vi "niScope Measure Dead Time.vi"(2 "error in":errorcluster, 3 "min sample rate":dbl=10000000.0 caption="Min. Sample Rate" step=1000000.0 format="%.3p", 4 "resource name":refnum<k15>="DAQ::1" caption="Resource Name") -> (0 "error out":errorcluster {"code" format="%.0x"}, 1 "Observed DeadTime":dbl)   [LabVIEW 2015]
doc: "Example: Measurement Library\n\nRecommended Input Signal: 100 kHz, 8 Vpp, sine wave\n\nDevices Supported: Refer to NI Example Finders\n\nLabVIEW Description:\n\nThis example illustrates fetching scalar measurements from NI-SCOPE, such as period and rise time calculations. \n\nSome common horizontal and vertical parameters are configured for the digitizer. The property node is used to set the reference level units, and the low, middle and high reference levels. For more information about measurement library parameters, see the NI-SCOPE VI Reference Help file. \n\nAfter the Read VI is called to acquire a waveform, the Fetch Measurement Stats VI is used to perform the desired scalar measurement analysis on the waveform. NI-SCOPE keeps a history of each measurement's results, which allows it to retrieve the statistics computed over multiple acquisitions. These statistics include the mean, standard deviation, min, max and number of acquisitions used in the statistics. The statistics are updated once per acquisition when the measurement is fetched. The Clear Stats VI clears this history."
uses:
  <instrlib>/niScope/Controls/niScope vertical coupling.ctl
  <instrlib>/niScope/Controls/niScope trigger source.ctl
  <instrlib>/niScope/Controls/niScope trigger coupling.ctl
  <instrlib>/niScope/Controls/niScope scalar measurement.ctl
  <instrlib>/niScope/Controls/niScope array measurement.ctl
  <instrlib>/niScope/Configure/Trigger/niScope Configure Trigger Edge.vi
  <instrlib>/niScope/Acquire/niScope Multi Read Cluster.vi
  <instrlib>/niScope/Measurements/niScope Multi Fetch Measurement Stats.vi
panel:
  out "Waveform Chart":u32(graph)
  out "x-y 2":u32
  out "x-y":u32
  out "Observed FallTime Ch 1":dbl format="%^.2e"
  out "Observed FallTime Ch 0":dbl format="%^.2e"
  out "Ch 0 - Fall Time":T1 {"scalar result" format="%^.2e"; "mean" format="%^.2e"; "stdev" format="%^.2e"; "min" format="%^.2e"; "max" format="%^.2e"; "num in stats" format="%^.2e"}
  out "Ch 1 - Fall Time":T1 {"scalar result" format="%^.2e"; "mean" format="%^.2e"; "stdev" format="%^.2e"; "min" format="%^.2e"; "max" format="%^.2e"; "num in stats" format="%^.2e"}
  out "Observed RiseTime Ch 1":dbl format="%^.2e"
  out "Observed RiseTime Ch 0":dbl format="%^.2e"
  out "Ch 0 - Rise Time":T1 {"scalar result" format="%^.2e"; "mean" format="%.2e"; "stdev" format="%.2e"; "min" format="%.2e"; "max" format="%.2e"; "num in stats" format="%.2e"}
  out "Ch 1 - Rise Time":T1 {"scalar result" format="%.2e"; "mean" format="%.2e"; "stdev" format="%.2e"; "min" format="%.2e"; "max" format="%.2e"; "num in stats" format="%.2e"}
  out "Fall Time Measurements":T2(array[cluster]) caption="stats" {"max" format="%^.2e"; "min" format="%^.2e"; "stdev" format="%^.2e"; "mean" format="%^.2e"; "scalar result" format="%^.2e"}
  out "Rise Time Measurements":T2(array[cluster]) caption="stats" {"max" format="%^.2e"; "min" format="%^.2e"; "stdev" format="%^.2e"; "mean" format="%^.2e"; "scalar result" format="%^.2e"}
  out "DeadTime Measurements":T2(array[cluster]) caption="stats" {"max" format="%.2p"; "min" format="%.2p"; "stdev" format="%.2p"; "mean" format="%.2p"; "scalar result" format="%.2p"}
  in  "stop":bool
  in  "Reference Level Units":i32(ring)=1 items=["Voltage", "Percentage"]
  in  "high reference":dbl=90.0 caption="High Ref." format="%.3f"
  in  "mid reference":dbl=50.0 caption="Mid Ref." format="%.3f"
  in  "low reference":dbl=10.0 caption="Low Ref." format="%.3f"
  out "Acquisition Graph":T3(graph)=[{"relativeInitialX"=-5.1119996754778185e-05, "xIncrement"=1e-07, "wfm"=[-4.06403104547644, -4.117707957106177, -4.163333331991453, -4.19755236315541, -4.198223324550781, -4.158636602223851, -4.110327381757088, -4.047927971987519, -3.976135102682747, -3.8835424301214516, -3.782898220815696, -3.6815830501145683, -3.539339234295767, -3.39508253429085, -3.226671224052552, -3.067653373349458, -2.8844809124129824, -2.7019794128718786, -2.5087425310048275, -2.302757382625714, -2.0759724309900776, -1.8491874793544412, -1.6351507942308672, -1.382869309571106, -1.1648068560753018, -0.8991061435081065, -0.6682954235002398, -0.4307750895386562, -0.1818484118557535, 0.0603686518734321, 0.3012437928118743, 0.5488285477040336, 0.7796392677119002, 1.03527555934852, 1.2566928198211826, 1.4888454626197927, 1.7015402249526232, 1.9175897942623124, 2.139678016130347, 2.3315729752066545, 2.5456096603302285, 2.701943665451836, 2.904574006854091, 3.036082440346945, 3.202480866399128, 3.3380150682642125, 3.459459080826491, 3.5607742515276186, 3.6681280747870915, 3.7426047896733508, 3.81305573618738, 3.874113223166205, 3.921751482237596, 3.9593253203784116, 3.9794541622395627, 3.9412093627033755, 3.8908872580504976, 3.842578037583735, 3.7748109366511926, 3.698321337578818, 3.6017028966452926, 3.4997167645487934, 3.3742469836142845, 3.225293553841766, 3.083720699418336, 2.9213480417383835, 2.7522657701047137, 2.5382290849811397, 2.3563985468354076, 2.1249168654321693, 1.9196026784484275, 1.692817726812791, 1.4506006630836055, 1.2278414798201993, 0.9809276863234118, 0.7152269737562165, 0.49515163607429713, 0.23079284629784524, 0.00333693326683715, -0.2529703197651543, -0.503909881634172, -0.7575332890846767, -0.9876730476971716, -1.2104322309605777, -1.4519783332943916, -1.7116403933032416, -1.9511736114509404, -2.1538039528531954, -2.404743514722213, -2.569129056588281, -2.7791399733396247, -2.9797574305557646, -3.1602460459107533, -3.3239606263814494, -3.4816365542938, -3.625222292903345, -3.730563231976703, -3.845968591980636, -3.944599917100277, -4.0090122110559605, -4.0774502733838744, -4.127101416641381, -4.175410637108143, -4.20560389989987, -4.180778328271117, -4.14655929710716, -4.092882385477424, -4.0271281687309965, -3.9519804924493656, -3.860058781283442, -3.760085533373058, -3.6332738296478055, -3.497739627782721, -3.352141004987061, -3.1911102700978518, -3.01733126869658, -2.8435522672953084, -2.6496444240328856, -2.4376206230954267, -2.2356612430885434, -2.0122310984297656, -1.792826722143218, -1.5385323532973416, -1.3218118225922808, -1.088988218398299, -0.8521388458320871, -0.6025412067538127, -0.35227260628016666, -0.1281715002260171, 0.10934883373556659, 0.3616303183953278, 0.6051893049152568, 0.83465810213238, 1.1017007374903187, 1.3157374226138927, 1.524406416574493, 1.779371746815741, 1.9612022849614732, 2.187316275201738, 2.3933014235808514, 2.5711061933543533, 2.7509238473139703, 2.940134960808791, 3.0937851203489117, 3.2420675887260586, 3.370892176637426, 3.4862975366413593, 3.596335205482319, 3.69899229897419, 3.773469013860449, 3.831171693862416, 3.885519566887524, 3.926448212005198, 3.960667243169155, 3.964693011541385, 3.924435327819083, 3.880822837119922, 3.8298297710716724, 3.753340171999298, 3.680876341299154, 3.582245016179513, 3.471536385943182, 3.338686029659584, 3.1951002910500392, 3.0280309036024846, 2.863645361736417, 2.6891953989397734, 2.510048706375528, 2.289302407298237, 2.066543224034831, 1.8598871142603457, 1.6431665835552849, 1.383504523546435, 1.1560486105154268, 0.9171863537630998, 0.6608791007311083, 0.4260426123510115, 0.1757740118773654, -0.06375920627033338, -0.28920223511522636, -0.5730189053574577, -0.8105392393190414, -1.0648336081649177, -1.3117474016617052, -1.5600031179492362, -1.778736532840412, -2.0122310984297656, -2.2309645133209415, -2.43493677751394, -2.648302501242142, -2.844894190086052, -3.0320924193947576, -3.1911102700978518, -3.3648892714991234, -3.5245780835975893, -3.6547445942997, -3.766124185931403, -3.8593878198880702, -3.9539933766354807, -4.025786245940253, -4.094895269663539, -4.145888335711788, -4.183462173852604, -4.210971591062844, -4.172726791526657, -4.137165837571956, -4.082817964546848, -4.010354133846704, -3.9338645347743295, -3.8399299394222908, -3.7245245794183575, -3.609790180809796, -3.4608367510372773, -3.313896205450874, -3.144813933817204, -2.971705893811304, -2.78517862589797, -2.5812063617049716, -2.3926662096055225, -2.173261833318975, -1.9538574570324272, -1.7203628914430737, -1.4929069784120657, -1.257399528636597, -1.036653229559306, -0.7883975132717751, -0.549535256519448, -0.31134396116249263, -0.05839151510735974, 0.1610128611791879, 0.4374489560723305, 0.6709435216616839, 0.9037671258556657, 1.1473261123755947, 1.367401450057514, 1.5921735175070353, 1.8290228900732473, 2.0128663124050945, 2.2403222254361026, 2.430875261721667, 2.6408861784730107, 2.8046007589437068, 2.9803926445310935, 3.138739533838816, 3.272931812913157, 3.3990725552430376, 3.5131359924562275, 3.621160777111072, 3.708385758509394, 3.7821915120002814, 3.8472747673513368, 3.8975968720042147, 3.9365126329357736, 3.9707316640997306, 3.9526157064246945, 3.915041868283879, 3.8680745706078596, 3.814397658978123, 3.7345532529288903, 3.650683078507427, 3.5426582938525826, 3.432620625011623, 3.2990993073326536, 3.1608812598860823, 2.999850524996873, 2.831439214758575, 2.637531371496152, 2.453687949164305, 2.2342835728777573, 2.02293073333567, 1.8109069323982112, 1.588147749134805, 1.355995106336195, 1.1117651584208943, 0.8749157858546823, 0.6118989188689739, 0.38175916025647894, 0.11404556350316852, -0.12213284766767174, -0.3851497146533802, -0.6528633114066906, -0.8709257649024948, -1.111800905840937, -1.346637394221034, -1.6210606049280614, -1.8203361393534578, -2.059198396105785, -2.28933815471828, -2.5020329170511104, -2.700637490081135, -2.896558217529673, -3.0750339486985467, -3.2400904519599862, -3.402463109639939, -3.559468076156918, -3.6742024747654796, -3.791620718955528, -3.8909230054705404, -3.9680835659382865, -4.045915087801404, -4.100262960826512, -4.147230258502532, -4.190842749201693, -4.206945822690614, -4.168030061759055, -4.127101416641381, -4.064702006871812, -3.9935800989624113, -3.9083680017502047, -3.8130914836074226, -3.7057376603479497, -3.5782549952273257, -3.425275797082577, -3.2763223673100583, -3.1139497096301056, -2.935473978461232, -2.728817868686747, -2.5677871337975375, -2.3423441049526446, -2.132333188201301, -1.9015224681934342, -1.6760794393485412, -1.45130737189902, -1.2231804974726401, -0.9635184374637902, -0.7199594509438612, -0.49049065372673795, -0.24693166720680892, -0.0006888351053930819, 0.2240832323441282, 0.48575817653909326, 0.725291394686792, 0.9386571184149943, 1.1862418733071536, 1.419736438896507, 1.6371279309969395, 1.8652548054233193, 2.0725818765931763, 2.287289523112122, 2.4818683277699165, 2.661015020334162, 2.8394907515030354, 3.0146116756950505, 3.1689327966305427, 3.3078218054724857, 3.4265819724532776, 3.544000216643326, 3.6500121171120554, 3.737237098510377, 3.8043332380475476, 3.8593520724680275, 3.910345138516277, 3.940538401308004, 3.9828089692164212, 3.9485899380524643, 3.908332254330162, 3.858010149677284, 3.790243048744742, 3.723817870602943, 3.630554236646276, 3.52588425896829, 3.409136976173613, 3.2762866198900156, 3.1239783831406385, 2.962947648251429, 2.7985621063853614, 2.5952608035877347, 2.4067206514882855, 2.19603877334157, 1.9907245863578282, 1.761255789140705, 1.5264193007606082, 1.2714539705193602, 1.0594301695819013, 0.7944004184100777, 0.5468156635179184, 0.3166759049054235, 0.06573634303640574, -0.1811774504603818, -0.42809124395716935, -0.6904371495475061, -0.9339961360674351, -1.1721874314243905, -1.410378726781346, -1.6418604081845842, -1.8753549737739377, -2.1007980026188307, -2.316176610533148, -2.544303484959528, -2.7321726756636053, -2.933461094275117, -3.101872404513415, -3.2823610198684037, -3.427288681268692, -3.5836226863902994, -3.696344200812746, -3.805710908258334, -3.905013194773346, -3.9902252919855528, -4.058663354313467, -4.113011227338575, -4.158636602223851, -4.198223324550781, -4.196881401760038, -4.156623718037736, -4.11099834315246, -4.042560280824546, -3.9815027938457206, -3.884884352912195, -3.7842401436064392, -3.6742024747654796, -3.552758462203201, -3.395753495686222, -3.2508258342859335, -3.067653373349458, -2.9025968700880185, -2.7086890268255956, -2.4966652258881368, -2.2967187300673686, -2.0806691607576795, -1.8485165179590695, -1.6304540644632652, -1.4043400742230006, -1.162123010493815, -0.9299703676952049, -0.6729921532678418, -0.4341298965155147, -0.17178399092517793, 0.05768480629194528, 0.30728244537021965, 0.5602348914253525, 0.789032727247104, 1.019172485859599, 1.2392478235415183, 1.4633489295956679, 1.690804842626676, 1.906854411936365, 2.1101557147339918, 2.330231052415911, 2.512732551957015, 2.701272704056464, 2.890483817551285, 3.0696305101155303, 3.199797020817641, 3.3467375664040446, 3.4695235017570667, 3.5701677110628225, 3.6654442292056046, 3.7432757510687225, 3.814397658978123, 3.8680745706078596, 3.9163837910746224, 3.955970513401553, 3.9774412780534476, 3.9371835943311453, 3.901622640376445, 3.8432489989791065, 3.7821915120002814, 3.7016761445556767, 3.6137802017619833, 3.496361957571935, 3.3789437133818865, 3.2534739324473776, 3.09311415895354, 2.9193351575522684, 2.744885194755625, 2.4959585170727223, 2.3402954733464867, 2.128271672409028, 1.9034996049595065, 1.661282541230321, 1.4365104737807997, 1.194293410051614, 0.9688503812067211, 0.7091883211978711, 0.47300991002703086, 0.2140188114135526, -0.03222402068786323, -0.2851764667429961, -0.5159871867508627, -0.793094243039377, -1.0098147737444378, -1.2634381811949424, -1.5224292798084207, -1.7418336560949683, -1.9706314919167198, -2.1900358682032675, -2.3993758235592395, -2.614754431473557, -2.81268804310821, -3.0032410793937743, -3.183729694748763, -3.349457159405574, -3.4923719366197474, -3.6151578719727695, -3.739285730116535, -3.8520072445389815, -3.9385612645419315, -4.015050863614306, -4.080134118965361, -4.126430455246009, -4.174739675712772, -4.2116425524582155, -4.185475058038719, -4.14253352873493, -4.086843732919078, -4.025115284544881, -3.9432579943095334, -3.8546910901204683, -3.748008228256367, -3.634615752438549, -3.4963977049919777, -3.348115236614831, -3.1783620035857894, -3.019344152882695, -2.835500730550848, -2.6288446207763627, -2.4470140826306306, -2.2155324012273923, -1.9934441793593578, -1.77001403470058, -1.5371904305065982, -1.312418363057077, -1.068859376537148, -0.8279842355987057, -0.5844252490787767, -0.3549564518616535, -0.11273938813246787, 0.12746479141060263, 0.3676689709536731, 0.5843895016587339, 0.8400257932953537, 1.0654688221402466, 1.3164083840092644, 1.5431933356449008, 1.7746750170481391, 1.9833440110087395, 2.2014064645045437, 2.4020239217206836, 2.591905996610876, 2.7690398049890064, 2.926715732901357, 3.095798004535027, 3.248106241284404, 3.38028563617263, 3.495690996176563, 3.6043867422267795, 3.6936246078112163, 3.773469013860449, 3.8412361147929914, 3.8861905282828957, 3.9338287873542868, 3.967376857122872, 3.95865435898304, 3.928461096191313, 3.880822837119922, 3.81708150455961, 3.751327287813183, 3.67148288176395, 3.589625591528602, 3.4654977333848365, 3.341369875241071, 3.184364908724092, 3.0233341738348827, 2.8596195933641866, 2.683156746381428, 2.489919864514377, 2.2819218319491483, 2.0672141854302026, 1.847809809143655, 1.633773124020081, 1.383504523546435, 1.1392745756311342, 0.8957155891112052, 0.6642339077079669, 0.4153072300250642, 0.17107728210976347, -0.07717843417776749, -0.32878895744215697, -0.5783865965204313, -0.8253003900172189, -1.0467176504898816, -1.3036958649172448, -1.5418871602742001, -1.788129992375616, -2.008876291452907, -2.2262677835533395, -2.461775233328808, -2.660379806358833, -2.8361716919462197, -3.047524531488307, -3.2078843049821444, -3.35952158033615, -3.5192103924346156, -3.6426672891830094, -3.7728337998851202, -3.8660974338417873, -3.953322415240109, -4.02847009152174, -4.092882385477424, -4.144546412921045, -4.186816980829462, -4.215668320830446, -4.176752559898887, -4.1297852622228675, -4.076108350593131, -4.017063747800421, -3.925812998029869, -3.8406009008176625, -3.7225116952322423, -3.5970419142977335, -3.4628496352233924, -3.2944383249850944, -3.1374333584681153, -2.962983395671472, -2.7777980505488813, -2.5798644389142282, -2.370524483558256, -2.1692360649467446, -1.94312207470648, -1.7277434667921625, -1.4888812100398354, -1.2594124128227122, -1.0171953490935266, -0.7696105942013673, -0.5502062179148197, -0.31134396116249263, -0.04564324859529734, 0.1992576607153751, 0.44617145421216264, 0.6783240970107727, 0.9138315467862412, 1.1359197686542757, 1.3848464463371783, 1.615657166345045, 1.811577893793583, 2.0450724593829364, 2.2342835728777573, 2.4449654510244727, 2.649608676612843, 2.7985621063853614, 2.981734567321837, 3.142765302211046, 3.2742737357039005, 3.407124091987498, 3.5292390659451485, 3.627870391064789, 3.7184501794399694, 3.7815205506049097, 3.84861669014208, 3.900951678981073, 3.9459060924709775, 3.970060702704359, 3.9526157064246945, 3.913028984097764, 3.864719763631001, 3.8043332380475476, 3.7291855617659166, 3.646657310135197, 3.548025985015556, 3.421214281290304, 3.3017831529141404, 3.140752418024931, 2.9917989882524125, 2.8233876780141145, 2.635518487310037, 2.4268494933494367, 2.2470318393898197, 2.0061566984513775, 1.7867523221648298, 1.556612563552335, 1.339892032847274, 1.0748622816754505, 0.8427096388768405, 0.5931119997985661, 0.34552724490640685, 0.09190383745590225, -0.13890688255196437, -0.40393663372378796, -0.6266958169871941, -0.9111834486247972, -1.139310323051177, -1.376159695617389, -1.6297831030678935, -1.8498584407498129, -2.063224164478015, -2.3054412282072008, -2.5161231063539162, -2.7160696021746844, -2.896558217529673, -3.081072601256892, -3.2488129500998184, -3.406488878012169, -3.546048848249484, -3.686950741277542, -3.7949755259323865, -3.893606851052027, -3.980160871054977, -4.0499408561736345, -4.112340265943203, -4.151926988270134, -4.189500826410949, -4.20560389989987, -4.157965640828479, -4.119720841292292, -4.057992392918095, -3.9955929831485264, -3.905013194773346, -3.805710908258334, -3.684937857091427, -3.5554423077846877, -3.4346692566177808, -3.2669289077748545, -3.0998595203273, -2.924067634739913, -2.730830752872862, -2.546316369145643, -2.323557185882237, -2.1061656937818043, -1.8820645877276547, -1.6680279026040807, -1.4251398774795234, -1.2157999221235514, -0.9635184374637902, -0.7139207983855158, -0.4576135453535244, -0.22680282534565777, -0.012095178826712072, 0.27037956862477586, 0.481732408166863, 0.7373686998034827, 0.9842824933002703, 1.1976482170284726, 1.4526135472697206, 1.6559148500673473, 1.8786740333307534, 2.096065525431186, 2.3067474035779014, 2.498642362654209, 2.6838277077768, 2.862974400341045, 3.026688980811741, 3.1783262561657466, 3.309834689658601, 3.4386592775699683, 3.555406560364645, 3.648670194321312, 3.7358951757196337, 3.8063461222336628, 3.865390725026373, 3.9143709068885073, 3.953286667820066, 3.9781122394488193, 3.9459060924709775, 3.908332254330162, 3.8566682268865407, 3.7821915120002814, 3.7117405654862523, 3.6204898157157004, 3.52588425896829, 3.4057821691967547, 3.268906044540927, 3.1165978077915497, 2.949528420343995, 2.783800955687184, 2.5751319617265835, 2.3886046938132495, 2.1785937770619057, 1.957176516589243, 1.7471655998378992, 1.5237354551791213, 1.2620605109841563, 1.0292369067901745, 0.7850069588748738, 0.5515123932855204, 0.29520514025352895, 0.04426557838451117, -0.22344801836879924, -0.45023297000443563, -0.6964758021058515, -0.943389595602639, -1.1782260839827359, -1.4392300667823292, -1.6640021342318505, -1.933728615171276, -2.1054947323864326, -2.3356344909989275, -2.5563807900762185, -2.7657207454321906, -2.944196476601064, -3.129381821723655, -3.2937673635897227, -3.4507723301067017, -3.5782549952273257, -3.7090924673248082, -3.817117251979653, -3.9157485770992935, -3.9976058673346415, -4.058663354313467, -4.1183789185015485, -4.167359100363683, -4.202249092923012, -4.192855633387808, -4.1546108338516206, -4.102946806407999, -4.045244126406033, -3.9613739519845694, -3.8775037775631063, -3.782898220815696, -3.6701767063932493, -3.531958658946678, -3.3870309975463897, -3.236064683587756, -3.065640489163343, -2.901254947297275, -2.700637490081135, -2.482575036585331, -2.2792737337877043, -2.059198396105785, -1.8424778654007241, -1.6002608016715385, -1.360056622128468, -1.1372974388650618, -0.8944094137405045, -0.654205234197434, -0.4361427807016298, -0.19124187139095739, 0.05432999931508675, 0.3166759049054235, 0.5602348914253525, 0.8158711830619723, 1.0218563314410858, 1.2613895495887846, 1.5076323816902004, 1.7223400282091461, 1.9404024817049503, 2.1517553212470375, 2.3503598942770623, 2.5382290849811397, 2.7167048161500134, 2.8938386245281436, 3.06157897337107, 3.2105324031435885, 3.3447246822179295, 3.4748911929200403, 3.584928861761, 3.6768505729269236, 3.7473015194409527, 3.823791118513327, 3.8734422617708333, 3.9210805208422244, 3.96268012735527, 3.9734155096812174, 3.9344997487496585, 3.8935711036319844, 3.835197462234646, 3.771456129674334, 3.6949665306019597, 3.5956642440869473, 3.4883104208274744, 3.3588148715207353, 3.229990283609368, 3.072314355697017, 2.9092707366216928, 2.737504619406536, 2.5429258147487417, 2.3020506738102995, 2.10948475333862, 1.8920932612381876, 1.6780565761146136, 1.4445620105252601, 1.2244866728433408, 0.9675084584159777, 0.7179108193377033, 0.4777066397946328, 0.19254804676165804, -0.03692075045546517, -0.27377012302167714, -0.5059227658202872, -0.7669267486198805, -1.0151824649074115, -1.2433093393337913, -1.4868683258537203, -1.7431755788857117, -1.9525155342416838, -2.184668177040294, -2.3966919779777527, -2.603348087752238, -2.8006107379915193, -2.997202426835429, -3.158233161724638, -3.3239606263814494, -3.491030013829004, -3.6191836403449997, -3.7406276529072784, -3.8520072445389815, -3.932522611983586, -4.014379902218934, -4.081476041756105, -4.134481991990469, -4.176081598503515, -4.208958706876729, -4.181449289666489, -4.143875451525673, -4.090198539895937, -4.025786245940253, -3.944599917100277, -3.853349167329725, -3.7560597650008276, -3.6238803701126017, -3.4970686663873494, -3.329328317544423, -3.1736652738181874, -3.007937809161376, -2.8200686184572987, -2.630186543567106, -2.4248723565833643, -2.218887208204251, -1.997469947731588, -1.7726978802820668, -1.5418871602742001, -1.3050377877079882, -1.0628207239788026, -0.8226165444357321, -0.5703350597759709, -0.34958876069867983, -0.10938458115560934, 0.13216152117820457, 0.365656086767558, 0.6246471853810363, 0.8541159825981595, 1.1164618881884962, 1.315066461218521, 1.5686898686690256, 1.7753459784435108, 1.9940793933346868, 2.209458001249004, 2.3933014235808514, 2.6053252245183103, 2.7777623031288385, 2.9555670729023404, 3.104520502674859, 3.252802971052006, 3.3856533273356035, 3.5111231082701124, 3.6137802017619833, 3.69899229897419, 3.7687722840928473, 3.839894192002248, 3.8888743738643825, 3.935841671540402, 3.9687187799136154, 3.960667243169155, 3.928461096191313, 3.8794809143291786, 3.8211072729318403, 3.741933828277979, 3.6721538431593217, 3.571509633853566, 3.4534204282681458, 3.3353312226827256, 3.193087406863924, 3.0448049384867772, 2.8569357477826998, 2.672421364055481, 2.4731458296300843, 2.289302407298237, 2.0517820733366534, 1.8665967282140628, 1.620353896112647, 1.3781368323834613, 1.1493389965617098, 0.898399434692692, 0.6575242937542498, 0.399875117931515, 0.1610128611791879, -0.10670073557412252, -0.3435501081403345, -0.5998573611723259, -0.8232875058311038, -1.0762399518862367, -1.3392568188719451, -1.555977349577006, -1.7941686449339613, -2.022295519360341, -2.2510933551820926, -2.4537236965843476, -2.673799034266267, -2.8724036072962917, -3.0434987631160766, -3.215935841726605, -3.3783084994065575, -3.5286038519698195, -3.6607832468580455, -3.7701499543036334, -3.871465125004761, -3.9613739519845694, -4.033166821289342, -4.094224308268167, -4.151256026874762, -4.183462173852604, -4.20560389989987, -4.172726791526657, -4.130456223618239, -4.075437389197759, -4.007670288265217, -3.930509727797471, -3.8312074412824586, -3.7158020812785253, -3.5896613389486447, -3.454798098478932, -3.302489861729555, -3.1280398989329115, -2.9569447431131266, -2.7777980505488813, -2.5885869370540604, -2.386627557047177, -2.1699070263421163, -1.9464768816833384, -1.7277434667921625, -1.4848554416676052, -1.2466641463106498, -1.0239049630472437, -0.7857136676902883]}]
  in  "min record length":i32=1024 caption="Min. Record Length"
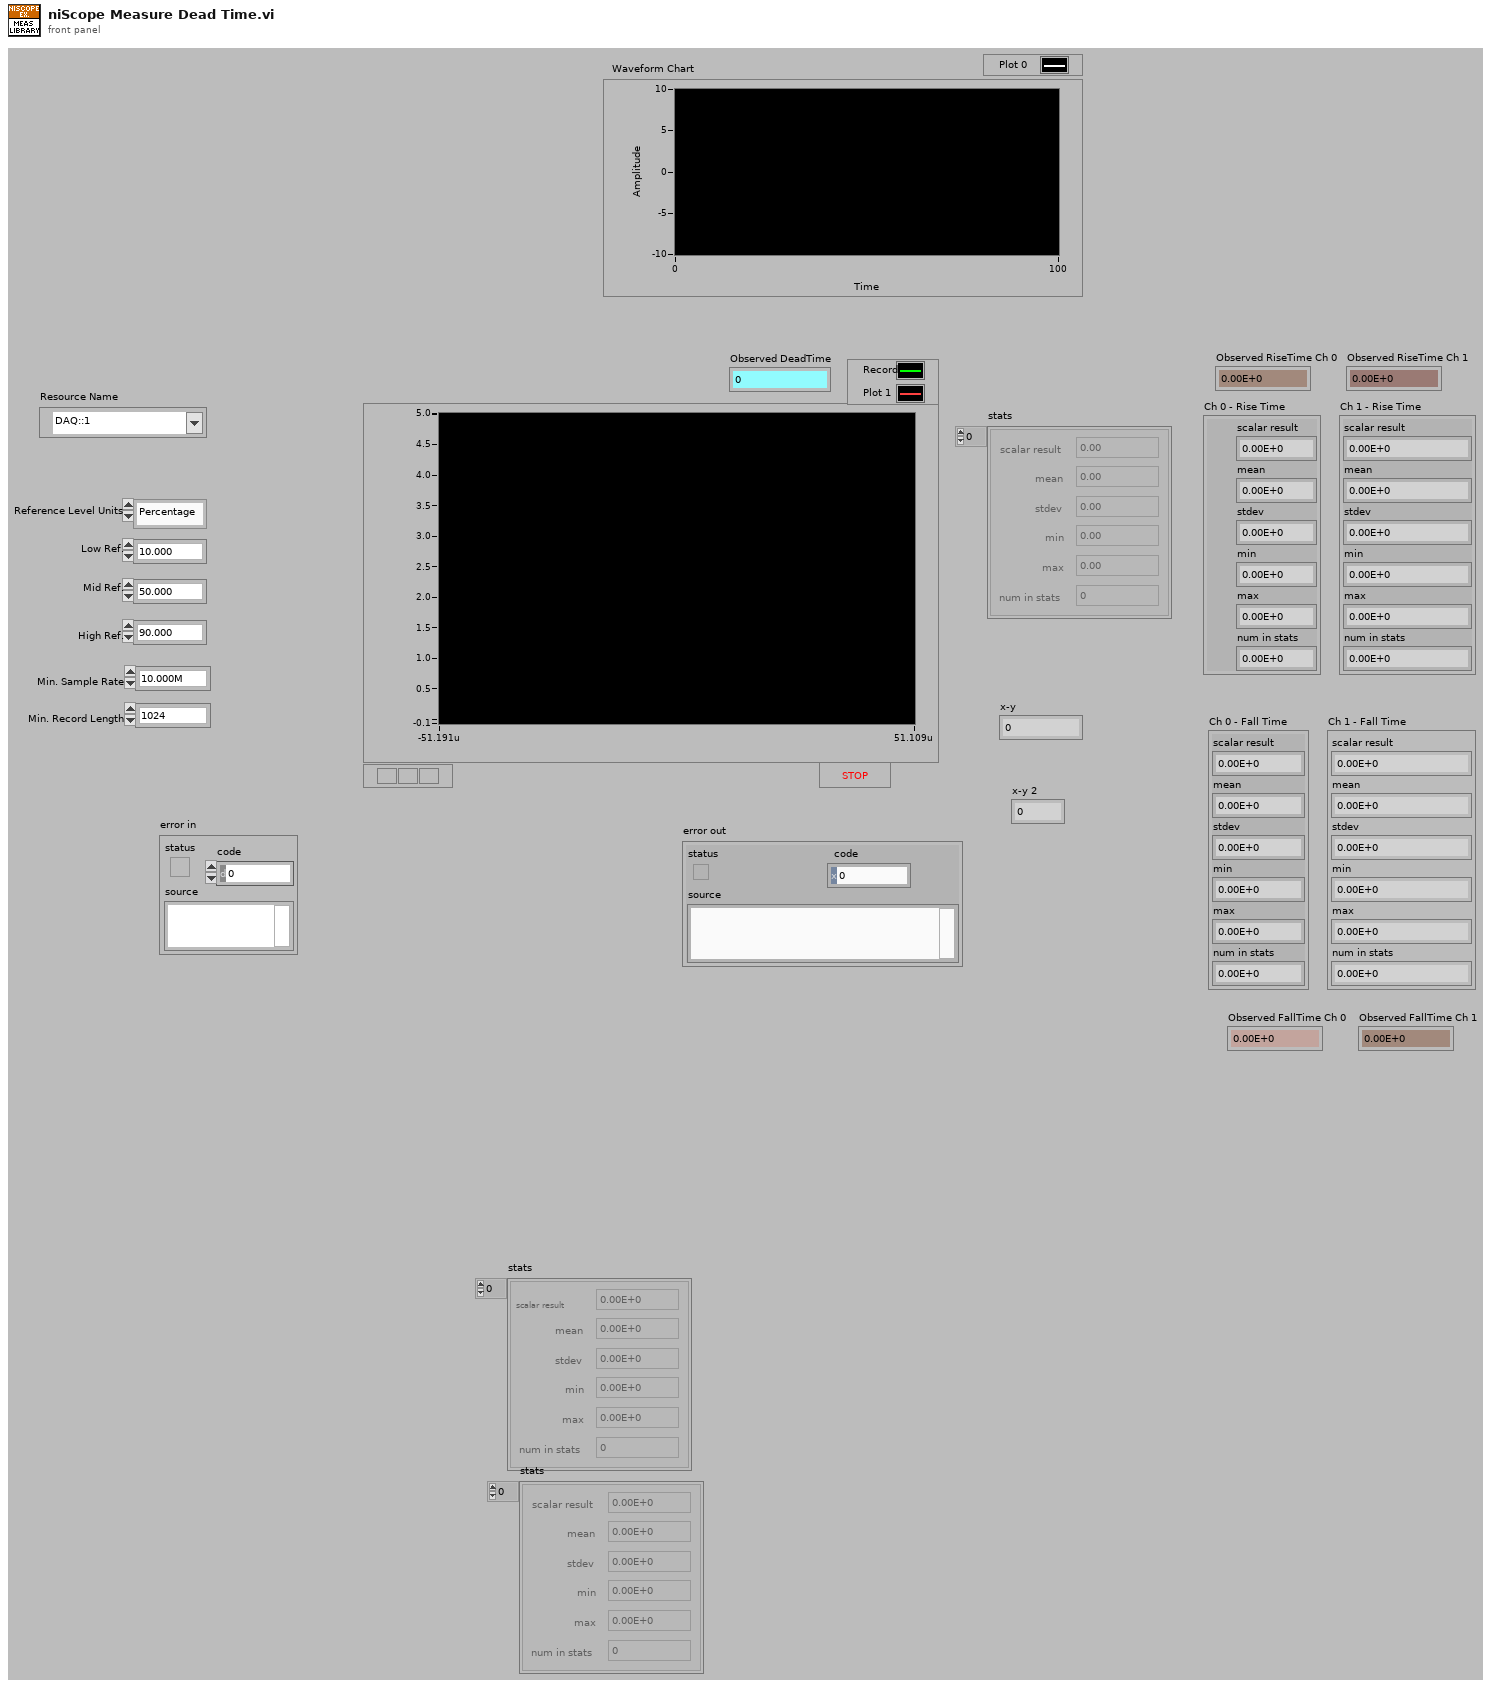
[diagram p1: front panel]
types:
  T1 = cluster{"scalar result":dbl, "mean":dbl, "stdev":dbl, "min":dbl, "max":dbl, "num in stats":i32}
  T2 = cluster{"scalar result":dbl, "mean":dbl, "stdev":dbl, "min":dbl, "max":dbl, "num in stats":i32}[]
  T3 = cluster{"relativeInitialX":dbl, "xIncrement":dbl, "wfm":dbl[]}[]
  T4 = typedef "niScope trigger coupling.ctl" = u16
  T5 = typedef "niScope trigger source.ctl" = string
  T6 = typedef "niScope vertical coupling.ctl" = i32
  T7 = typedef "niScope scalar measurement.ctl" = i32
  T8 = typedef "niScope array measurement.ctl" = i32
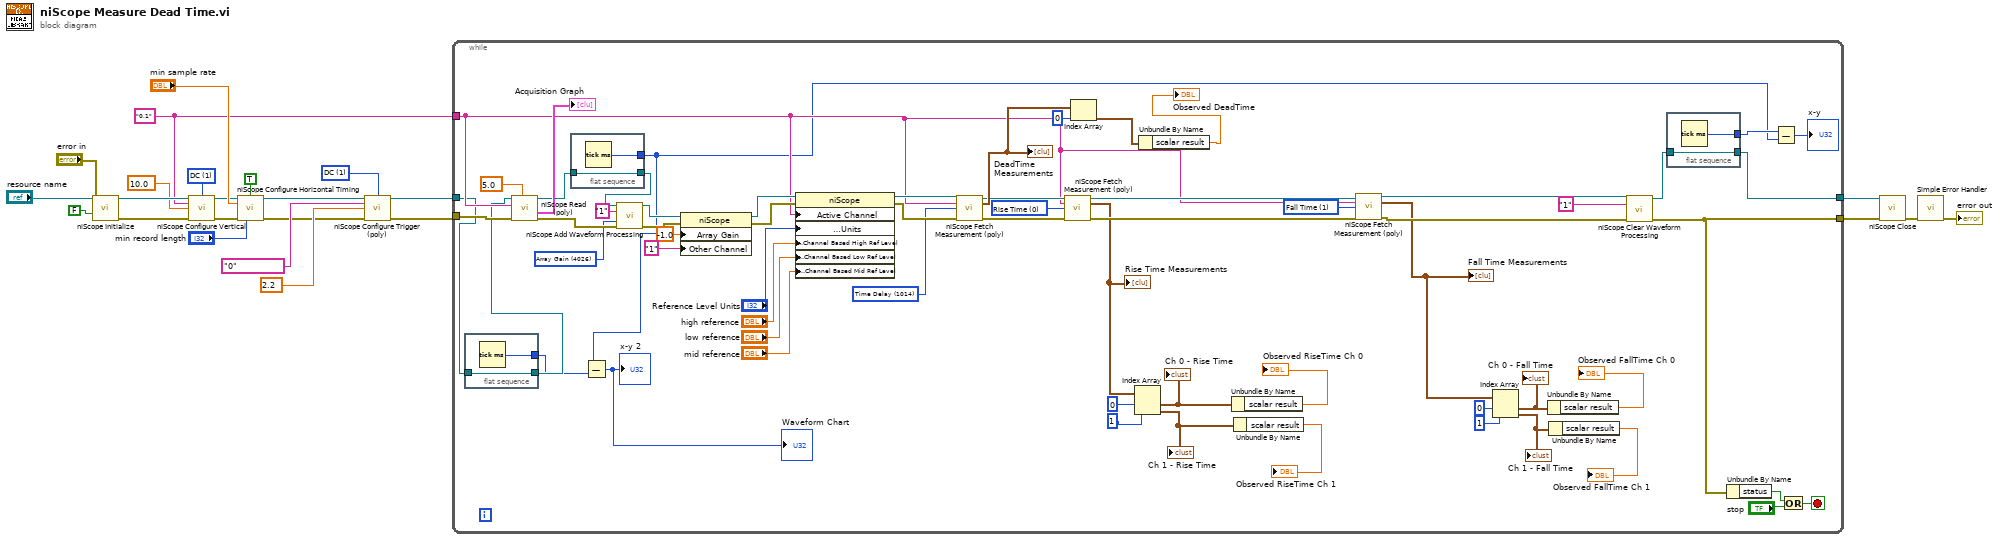
[diagram p0: block diagram]
diagram:
  w7 = T4 1 items=["AC"=0, "DC"=1, "HF Reject"=3, "LF Reject"=4, "AC Plus HF Reject"=1001] ("trigger coupling 2")
  w9 = "0,1" ("input channel")
  w10 = T6 1 items=["AC", "DC", "Ground"] ("vertical coupling")
  n1 = call <instrlib>:"niScope Initialize.vi"("resource name"="resource name", "reset device"=FALSE, "error in"="error in") -> ("instrument handle"=w18:refnum<k15>, "error out"=w17:errorcluster)  [unwired: 11 in]
  n2 = call <instrlib>:"niScope Configure Vertical.vi"("instrument handle"=w18, "vertical coupling"=w10, "channels"=w9, "vertical range"=10.0, "error in"=w17) -> ("instrument handle out"=w12:refnum<k15>, "error out"=w11:errorcluster)  [unwired: 9 in]
  n3 = call <instrlib>:"niScope Configure Horizontal Timing.vi"("instrument handle"=w12, "enforce realtime"=TRUE ("Enforce Realtime"), "min sample rate"="min sample rate", "error in"=w11, "min record length"="min record length") -> ("instrument handle out"=w5:refnum<k15>, "error out"=w4:errorcluster)  [unwired: 9 in]
  n4 = call-poly <instrlib>:"niScope Configure Trigger (poly).vi"("instrument handle"=w5, "trigger coupling"=w7, "trigger source"=T5 "0" ("Source"), "trigger level"=2.2, "error in"=w4) -> ("instrument handle out"=w2:refnum<k15>, "error out"=w3:errorcluster)  [unwired: 9 in]
  n5 = while {
    tunnel: [w65] -> w20
    tunnel: [w32] -> w19
    tunnel: w9 -> [w50]
    tunnel: w2 -> [w29]
    tunnel: w3 -> [w74]
    stop <- w78 stop-if-true
    w51 = T7 1 items=["None"=4000, "Frequency"=2, "Average Frequency"=1016, "FFT Frequency"=1008, "Period"=3, "Average Period"=1015, "Rise Time"=0, "Fall Time"=1, "Rising Slew Rate"=1010, "Falling Slew Rate"=1011, "Overshoot"=18, "Preshoot"=19, "Voltage RMS"=4, "Voltage Cycle RMS"=16, "AC Estimate"=1012, "FFT Amplitude"=1009, "Voltage Average"=10, "Voltage Cycle Average"=17, "DC Estimate"=1013, "Voltage Max"=6, "Voltage Min"=7, "Voltage Peak-to-Peak"=5, "Voltage High"=8, "Voltage Low"=9, "Voltage Amplitude"=15, "Voltage Top"=1007, "Voltage Base"=1006, "Voltage Base-to-Top"=1017, "Negative Width"=11, "Positive Width"=12, "Negative Duty Cycle"=13, "Positive Duty Cycle"=14, "Integral"=1005, "Area"=1003, "Cycle Area"=1004, "Time Delay"=1014, "Phase Delay"=1018, "Low Ref Volts"=1000, "Mid Ref Volts"=1001, "High Ref Volts"=1002, "Volt. Hist. Mean"=2000, "Volt. Hist. Stdev"=2001, "Volt. Hist. Median"=2003, "Volt. Hist. Mode"=2010, "Volt. Hist. Max"=2005, "Volt. Hist. Min"=2006, "Volt. Hist. Peak-to-Peak"=2002, "Volt. Hist. Mean + Stdev"=2007, "Volt. Hist. Mean + 2 Stdev"=2008, "Volt. Hist. Mean + 3 Stdev"=2009, "Volt. Hist. Hits"=2004, "Volt. Hist. New Hits"=2011, "Time Hist. Mean"=3000, "Time Hist. Stdev"=3001, "Time Hist. Median"=3003, "Time Hist. Mode"=3010, "Time Hist. Max"=3005, "Time Hist. Min"=3006, "Time Hist. Peak-to-Peak"=3002, "Time Hist. Mean + Stdev"=3007, "Time Hist. Mean + 2 Stdev"=3008, "Time Hist. Mean + 3 Stdev"=3009, "Time Hist. Hits"=3004, "Time Hist. New Hits"=3011] ("scalar measurement")
    w52 = T7 0 items=["None"=4000, "Frequency"=2, "Average Frequency"=1016, "FFT Frequency"=1008, "Period"=3, "Average Period"=1015, "Rise Time"=0, "Fall Time"=1, "Rising Slew Rate"=1010, "Falling Slew Rate"=1011, "Overshoot"=18, "Preshoot"=19, "Voltage RMS"=4, "Voltage Cycle RMS"=16, "AC Estimate"=1012, "FFT Amplitude"=1009, "Voltage Average"=10, "Voltage Cycle Average"=17, "DC Estimate"=1013, "Voltage Max"=6, "Voltage Min"=7, "Voltage Peak-to-Peak"=5, "Voltage High"=8, "Voltage Low"=9, "Voltage Amplitude"=15, "Voltage Top"=1007, "Voltage Base"=1006, "Voltage Base-to-Top"=1017, "Negative Width"=11, "Positive Width"=12, "Negative Duty Cycle"=13, "Positive Duty Cycle"=14, "Integral"=1005, "Area"=1003, "Cycle Area"=1004, "Time Delay"=1014, "Phase Delay"=1018, "Low Ref Volts"=1000, "Mid Ref Volts"=1001, "High Ref Volts"=1002, "Volt. Hist. Mean"=2000, "Volt. Hist. Stdev"=2001, "Volt. Hist. Median"=2003, "Volt. Hist. Mode"=2010, "Volt. Hist. Max"=2005, "Volt. Hist. Min"=2006, "Volt. Hist. Peak-to-Peak"=2002, "Volt. Hist. Mean + Stdev"=2007, "Volt. Hist. Mean + 2 Stdev"=2008, "Volt. Hist. Mean + 3 Stdev"=2009, "Volt. Hist. Hits"=2004, "Volt. Hist. New Hits"=2011, "Time Hist. Mean"=3000, "Time Hist. Stdev"=3001, "Time Hist. Median"=3003, "Time Hist. Mode"=3010, "Time Hist. Max"=3005, "Time Hist. Min"=3006, "Time Hist. Peak-to-Peak"=3002, "Time Hist. Mean + Stdev"=3007, "Time Hist. Mean + 2 Stdev"=3008, "Time Hist. Mean + 3 Stdev"=3009, "Time Hist. Hits"=3004, "Time Hist. New Hits"=3011] ("scalar measurement")
    w66 = T8 4026 items=["None"=4000, "Last Acq. Histogram"=4001, "Multi Acq. Voltage Histogram"=4004, "Multi Acq. Time Histogram"=4005, "Multi Acq. Average"=4016, "Polynomial Interpolation"=4011, "Array Integral"=4006, "Derivative"=4007, "Inverse"=4008, "Multiply Channels"=4012, "Add Channels"=4013, "Subtract Channels"=4014, "Divide Channels"=4015, "Array Offset"=4025, "Array Gain"=4026, "Hanning Window"=4009, "Flat Top Window"=4010, "Hamming Window"=4020, "Triangle Window"=4023, "Blackman Window"=4024, "FIR Windowed Filter"=4021, "Bessel IIR Filter"=4022, "Butterworth IIR Filter"=4017, "Chebyshev IIR Filter"=4018, "FFT Phase Spectrum"=4002, "FFT Amp. Spectrum (Volts RMS)"=4003, "FFT Amp. Spectrum (dB)"=4019] ("array measurement")
    w75 = T7 1014 items=["None"=4000, "Frequency"=2, "Average Frequency"=1016, "FFT Frequency"=1008, "Period"=3, "Average Period"=1015, "Rise Time"=0, "Fall Time"=1, "Rising Slew Rate"=1010, "Falling Slew Rate"=1011, "Overshoot"=18, "Preshoot"=19, "Voltage RMS"=4, "Voltage Cycle RMS"=16, "AC Estimate"=1012, "FFT Amplitude"=1009, "Voltage Average"=10, "Voltage Cycle Average"=17, "DC Estimate"=1013, "Voltage Max"=6, "Voltage Min"=7, "Voltage Peak-to-Peak"=5, "Voltage High"=8, "Voltage Low"=9, "Voltage Amplitude"=15, "Voltage Top"=1007, "Voltage Base"=1006, "Voltage Base-to-Top"=1017, "Negative Width"=11, "Positive Width"=12, "Negative Duty Cycle"=13, "Positive Duty Cycle"=14, "Integral"=1005, "Area"=1003, "Cycle Area"=1004, "Time Delay"=1014, "Phase Delay"=1018, "Low Ref Volts"=1000, "Mid Ref Volts"=1001, "High Ref Volts"=1002, "Volt. Hist. Mean"=2000, "Volt. Hist. Stdev"=2001, "Volt. Hist. Median"=2003, "Volt. Hist. Mode"=2010, "Volt. Hist. Max"=2005, "Volt. Hist. Min"=2006, "Volt. Hist. Peak-to-Peak"=2002, "Volt. Hist. Mean + Stdev"=2007, "Volt. Hist. Mean + 2 Stdev"=2008, "Volt. Hist. Mean + 3 Stdev"=2009, "Volt. Hist. Hits"=2004, "Volt. Hist. New Hits"=2011, "Time Hist. Mean"=3000, "Time Hist. Stdev"=3001, "Time Hist. Median"=3003, "Time Hist. Mode"=3010, "Time Hist. Max"=3005, "Time Hist. Min"=3006, "Time Hist. Peak-to-Peak"=3002, "Time Hist. Mean + Stdev"=3007, "Time Hist. Mean + 2 Stdev"=3008, "Time Hist. Mean + 3 Stdev"=3009, "Time Hist. Hits"=3004, "Time Hist. New Hits"=3011] ("scalar measurement")
    n6 = flat-sequence {
      tunnel: w29 -> [w88]
      tunnel: [w88] -> w28
      tunnel: [w87] -> w27
      frame #0 {
        n7 = Tick Count (ms)() -> (millisecond timer value=w87:u32)
      }
    }
    n8 = call-poly <instrlib>:"niScope Read (poly).vi"("timeout"=5.0 ("Max.Time"), "error in"=w74, "channels"=w50, "instrument handle"=w28) -> ("error out"=w67:errorcluster, "waveform"=→"Acquisition Graph":T3, "instrument handle out"=w35:refnum<k15>)  [unwired: 4 in, 1 out]
    n9 = flat-sequence {
      tunnel: w35 -> [w92]
      tunnel: [w92] -> w34
      tunnel: [w91] -> w26
      frame #0 {
        n10 = Tick Count (ms)() -> (millisecond timer value=w91:u32)
      }
    }
    n11 = Subtract(x=w26, y=w27) -> (x-y=→"x-y 2" →"Waveform Chart":u32)
    n12 = call <instrlib>:"niScope Add Waveform Processing.vi"("instrument handle"=w34, "channels"="1", "array measurement"=w66, "error in"=w67) -> ("instrument handle out"=w72:refnum<k15>, "error out"=w73:errorcluster)  [unwired: 10 in]
    n13 = property class="niScope"(reference=w72, error in=w73, "Array Gain"=-1.0 ("Waveform Measurement:Array Gain"), "Other Channel"="1" ("Waveform Measurement:Other Channel")) -> (reference out=w69:refnum<k15>, error out=w68:errorcluster)
    n14 = property class="niScope"(reference=w69, error in=w68, "Active Channel"=w50, "Waveform Measurement:Reference Levels:Units"="Reference Level Units", "Waveform Measurement:Reference Levels:Channel Based High Ref Level"="high reference", "Waveform Measurement:Reference Levels:Channel Based Low Ref Level"="low reference", "Waveform Measurement:Reference Levels:Channel Based Mid Ref Level"="mid reference") -> (reference out=w80:refnum<k15>, error out=w81:errorcluster)
    n15 = call-poly <instrlib>:"niScope Fetch Measurement (poly).vi"("instrument handle"=w80, "channels"=w50, "scalar measurement"=w75, "error in"=w81) -> ("instrument handle out"=w58:refnum<k15>, "stats"=w62:T2, "error out"=w55:errorcluster)  [unwired: 9 in]
    "DeadTime Measurements" <- w62
    n16 = call-poly <instrlib>:"niScope Fetch Measurement (poly).vi"("instrument handle"=w58, "channels"=w50, "scalar measurement"=w52, "error in"=w55) -> ("instrument handle out"=w57:refnum<k15>, "stats"=w45:T2, "error out"=w54:errorcluster)  [unwired: 9 in]
    "Rise Time Measurements" <- w45
    n17 = Index Array(array=w62, index=0) -> (element=w60:T1)
    n18 = Index Array(array=w45, index #1=0 ("index"), index #2=1 ("index")) -> (element #1=w49:T1, element #2=w47:T1)
    "Ch 1 - Rise Time" <- w47
    "Ch 0 - Rise Time" <- w49
    n19 = Unbundle By Name(w60) -> ("scalar result"=→"Observed DeadTime":dbl)
    n20 = Unbundle By Name(w49) -> ("scalar result"=→"Observed RiseTime Ch 0":dbl)
    n21 = Unbundle By Name(w47) -> ("scalar result"=→"Observed RiseTime Ch 1":dbl)
    n22 = call-poly <instrlib>:"niScope Fetch Measurement (poly).vi"("instrument handle"=w57, "channels"=w50, "scalar measurement"=w51, "error in"=w54) -> ("instrument handle out"=w56:refnum<k15>, "stats"=w38:T2, "error out"=w53:errorcluster)  [unwired: 9 in]
    "Fall Time Measurements" <- w38
    n23 = Index Array(array=w38, index #1=0 ("index"), index #2=1 ("index")) -> (element #1=w42:T1, element #2=w41:T1)
    "Ch 1 - Fall Time" <- w41
    "Ch 0 - Fall Time" <- w42
    n24 = Unbundle By Name(w42) -> ("scalar result"=→"Observed FallTime Ch 0":dbl)
    n25 = Unbundle By Name(w41) -> ("scalar result"=→"Observed FallTime Ch 1":dbl)
    n26 = call <instrlib>:"niScope Clear Waveform Processing.vi"("instrument handle"=w56, "channels"="1", "error in"=w53) -> ("instrument handle out"=w33:refnum<k15>, "error out"=w65:errorcluster)  [unwired: 11 in]
    n27 = flat-sequence {
      tunnel: w33 -> [w90]
      tunnel: [w90] -> w32
      tunnel: [w89] -> w30
      frame #0 {
        n28 = Tick Count (ms)() -> (millisecond timer value=w89:u32)
      }
    }
    n29 = Unbundle By Name(w65) -> ("status"=w76:bool)
    n30 = Subtract(x=w30, y=w26) -> (x-y=→"x-y":u32)
    n31 = Or(x=w76, y="stop") -> (x .or. y?=w78:bool)
  }
  n32 = call <instrlib>:"niScope Close.vi"("instrument handle"=w19, "error in"=w20) -> ("error out"=w22:errorcluster)  [unwired: 13 in]
  n33 = call <vilib>:"Simple Error Handler.vi"("error in (no error)"=w22) -> ("error out"=→"error out":errorcluster)  [unwired: 4 in, 4 out]
